vi "Is Recieve Ready.vi"(8 "error in (no error)":errorcluster, 10 "Points to read":i32, 11 "RP Instrument in":refnum<class "RP Instrument.lvclass">) -> (0 "error out":errorcluster, 1 "Points in buffer":i32, 2 "Recieve Ready":bool, 3 "RP Instrument out":refnum<class "RP Instrument.lvclass">)   [LabVIEW 2019, in "RP Instrument.lvclass"]
uses:
  RP Instrument.lvclass
  RP Status Offsets.ctl
  RP Instrument.lvclass/RP Instrument.ctl
  RP Communicator/RP Communicator.lvclass
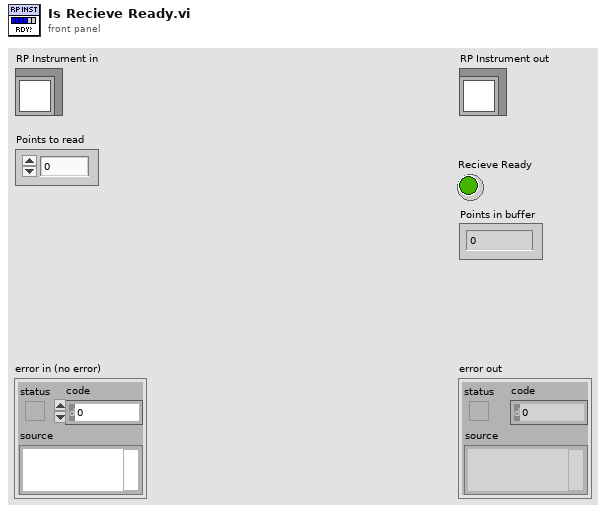
[diagram p1: front panel]
types:
  T1 = typedef "RP Status Offsets.ctl" = u16
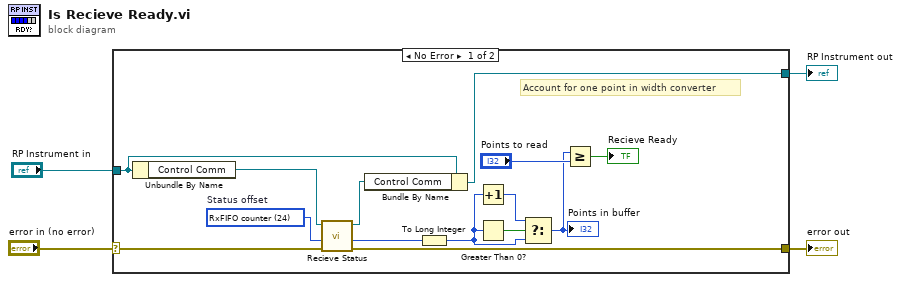
[diagram p0: block diagram]
diagram:
  n1 = case shown="No Error" "error in (no error)" {
    selector: "error in (no error)" -> [w12 w20]
    tunnel: [w11 w20] -> w3
    tunnel: [w14 w19] -> w1
    tunnel: "RP Instrument in" -> [w18 w19]
    frame No Error {
      w16 = T1 24 items=["Writer address"=0, "Record start position"=4, "Trig state etc."=8, "RxFIFO counter"=24, "TxFIFO counter"=28]  # Status offset
      # "Account for one point in width converter"
      n2 = Unbundle By Name(w18) -> ("Control Comm"=w17:refnum<class "RP Communicator.lvclass">)
      n3 = call-dynamic "Recieve Status.vi"("error in (no error)"=w12, "Status offset"=w16, "RP Communicator in"=w17) -> ("error out"=w11:errorcluster, "Status response"=w9:u32, "RP Communicator out"=w13:refnum<class "RP Communicator.lvclass">)  [unwired: 6 in]
      n4 = Bundle By Name(cluster=w18, "Control Comm"=w13) -> (w14:refnum<class "RP Instrument.lvclass">)
      n5 = To Long Integer(number=w9) -> (32bit integer=w6:i32)
      n6 = Increment(x=w6) -> (x+1=w7:i32)
      n7 = Greater Than 0?(x=w6) -> (x > 0?=w8:bool)
      n8 = Select(t=w7, s=w8, f=w6) -> (s? t:f=w5:i32)
      "Points in buffer" <- w5
      n9 = Greater Or Equal?(x=w5, y="Points to read") -> (x >= y?=→"Recieve Ready":bool)
    }
    frame Error {
    }
  }
  "error out" <- w3
  "RP Instrument out" <- w1
